vi "LoadDiagram.vi"(2 "SubPanel in":refnum<vi>, 3 "Code name":string) -> ()   [LabVIEW 2012]
panel:
  out "open?":bool
  out "error out":errorcluster
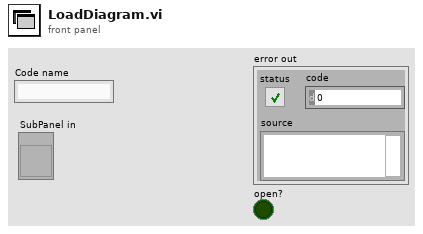
[diagram p1: front panel]
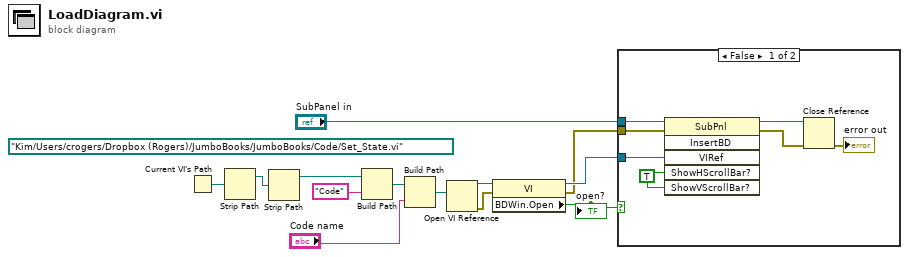
[diagram p0: block diagram]
diagram:
  (unwired) path "/Kim/Users/crogers/Dropbox (Rogers)/JumboBooks/JumboBooks/Code/Set_State.vi" ("vi path")
  n1 = Current VI's Path() -> (path=w9:path)
  n2 = Strip Path(path=w9) -> (stripped path=w8:path)  [unwired: 1 out]
  n3 = Strip Path(path=w8) -> (stripped path=w7:path)  [unwired: 1 out]
  n4 = Build Path(base path=w7, name or relative path="Code") -> (appended path=w11:path)
  n5 = Build Path(base path=w11, name or relative path="Code name") -> (appended path=w1:path)
  n6 = Open VI Reference(vi path=w1) -> (vi reference=w5:refnum<vi>, error out=w6:errorcluster)  [unwired: 5 in]
  n7 = property class="VI"(reference=w5, error in=w6) -> (reference out=w4:refnum<vi>, error out=w3:errorcluster, "BDWin.Open"=w2:bool)
  "open?" <- w2
  n8 = case shown="False" w2 {
    tunnel: "SubPanel in" -> [w20 _]
    tunnel: w4 -> [w15 _]
    tunnel: w3 -> [w14 _]
    frame False {
      w19 = TRUE ("ShowHScrollBar")
      n9 = invoke class="SubPnl" method="InsertBD"(reference=w20, error in=w14, "VIRef"=w15, "ShowHScrollBar?"=w19, "ShowVScrollBar?"=w19) -> (reference out=w18:refnum<vi>, error out=w16:errorcluster)  [unwired: 1 in, 4 out]
      n10 = Close Reference(reference=w18, error in (no error)=w16) -> (error out=→"error out":errorcluster)
    }
    frame True {
    }
  }
